vi "Missing VI Message.vi"(11 "Missing VI Type in":refnum<class "Missing VI Type.lvclass">) -> ()   [LabVIEW 2020, in "Peek Window.lvlib" / "Missing VI Type.lvclass"]
uses:
  Missing VI Type.lvclass
panel:
  out "VI Expected Path":path
  out "VI Full Qualified Name":string
  # "This VI is Missing. \nThe Block Diagram cannot be displayed."
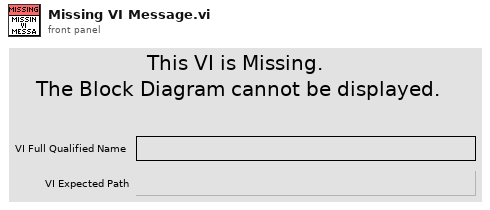
[diagram p1: front panel]
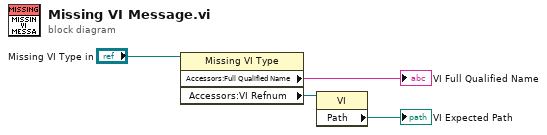
[diagram p0: block diagram]
diagram:
  n1 = property class="Missing VI Type"(reference="Missing VI Type in") -> ("Accessors:Full Qualified Name"=→"VI Full Qualified Name":string, "Accessors:VI Refnum"=w2:refnum<vi>)  [unwired: 1 in, 2 out]
  n2 = property class="VI"(reference=w2) -> ("Path"=→"VI Expected Path":path)  [unwired: 1 in, 2 out]
